vi "set request timeout.vi"(8 "error in (no error)":errorcluster, 10 "request timeout (ms)":i32, 11 "Nominal Client in":refnum<class "Nominal Client.lvclass">) -> (0 "error out":errorcluster, 3 "Nominal Client out":refnum<class "Nominal Client.lvclass">)   [LabVIEW 2020, in "Nominal Client.lvclass"]
uses:
  Nominal Client.lvclass
  Nominal Client.lvclass/Nominal Client.ctl
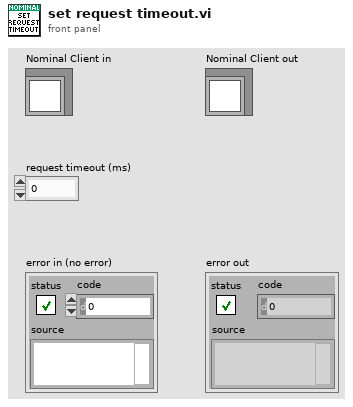
[diagram p1: front panel]
types:
  T1 = typedef "Nominal Client.lvclass/private_data.ctl" = cluster{"API Token":string, "workspace":refnum<class "workspace.lvclass">, "Available Workspaces":refnum<class "workspace.lvclass">[], "reqwest":refnum<class "reqwest.lvclass">, "timeout ms":i32}
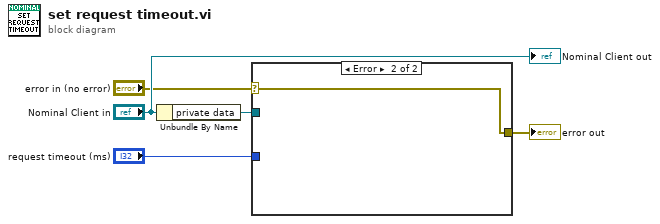
[diagram p0: block diagram]
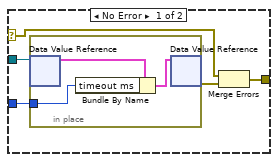
[diagram p2: hidden frame]
diagram:
  n1 = Unbundle By Name("Nominal Client in") -> ("private data"=w4:refnum<data-value>)
  n2 = case shown="Error" "error in (no error)" {
    selector: "error in (no error)" -> [w8 w14]
    tunnel: w4 -> [w10 _]
    tunnel: "request timeout (ms)" -> [w9 _]
    tunnel: [w6 w14] -> w1
    frame No Error {
      n3 = in-place {
        in-place-border: w9 -> [w12]
        n4 = in-place-dvr #1(w10) -> (w13:T1)  [unwired: 1 out]
        n5 = Bundle By Name(cluster=w13, "timeout ms"=w12) -> (w11:T1)
        n6 = in-place-dvr #1(w11) -> (w7:errorcluster)  [unwired: 1 out]
      }
      n7 = Merge Errors(w8, w7) -> (w6:errorcluster)
    }
    frame Error {
    }
  }
  "error out" <- w1
  "Nominal Client out" <- "Nominal Client in"
